vi "CRYFlatten SoundCard.vi"(11 "SoundCard":T1={"Name"="", "Analog I/O"=0, "Digital I/O"=0, "Channels"=2, "Dig Dev ID"=1, "N ports"=3, "Interface"=0, "Dig I/O Ports"=[{"port #"=1, "width"=8, "direction"=0}, {"port #"=2, "width"=8, "direction"=0}, {"port #"=3, "width"=8, "direction"=0}], "Interf settings"=[], "N interfs"=3, "udev SNs"=[], "udev enable"=FALSE, "Channel Array"=[], "Cal sequence"="", "SelectedIn"=0, "SelectedOut"=0, "SelectedTab"=0, "State"=FALSE, "Help"="", "Advanced"=FALSE, "In Audio Driver"=0, "Out Audio Driver"=0} {"Channel Array"."Coupling" items=["Default"=-1, "RSE"=10083, "NRSE"=10078, "Differential"=10106, "Pseudodifferential"=12529]; "Channel Array"."term config" items=["Default"=-1, "RSE"=10083, "NRSE"=10078, "Differential"=10106, "Pseudodifferential"=12529]; "Channel Array"."Anti-aliasing Factor (%fs)" format="%.2f"}) -> (3 "SoundCard flattened":string)   [LabVIEW 2013]
uses:
  Typedef Control/CRYHardware.ctl
  Typedef Control/CRYHardware Channel Info.ctl
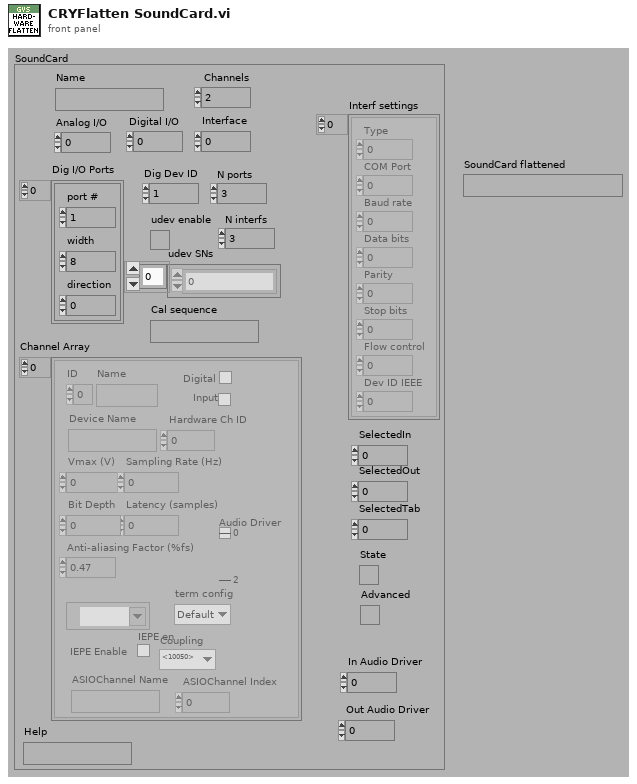
[diagram p1: front panel]
types:
  T1 = typedef "CRYHardware.ctl" = cluster{"Name":string, "Analog I/O":u16, "Digital I/O":u16, "Channels":u8, "Dig Dev ID":u8, "N ports":u8, "Interface":u32, "Dig I/O Ports":cluster{"port #":i16, "width":i16, "direction":i32}[], "Interf settings":cluster{"Type":u16, "COM Port":u8, "Baud rate":u32, "Data bits":u32, "Parity":u16, "Stop bits":u16, "Flow control":u16, "Dev ID IEEE":u8}[], "N interfs":i32, "udev SNs":i16[], "udev enable":bool, "Channel Array":T2[], "Cal sequence":string, "SelectedIn":u16, "SelectedOut":u16, "SelectedTab":u16, "State":bool, "Help":string, "Advanced":bool, "In Audio Driver":u16, "Out Audio Driver":u16}
  T2 = typedef "CRYHardware Channel Info.ctl" = cluster{"ID":i32, "Name":string, "Digital":bool, "Input":bool, "Device Name":string, "Hardware Ch ID":u8, "Vmax (V)":dbl, "Latency (samples)":dbl, "Sampling Rate (Hz)":u32, "Bit Depth":u32, "Anti-aliasing Factor (%fs)":sgl, "DAQmx Channel":tag, "term config":i32, "Coupling":i32, "IEPE en":bool, "ASIOChannel Name":string, "Audio Driver":u16, "ASIOChannel Index":u8}
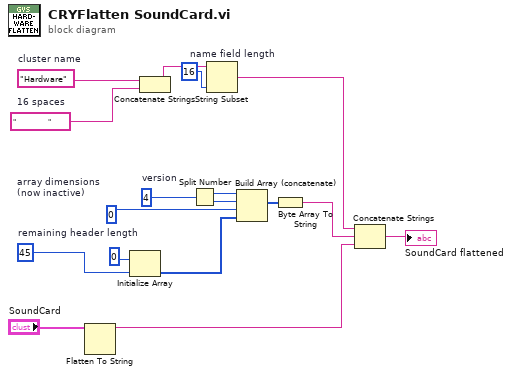
[diagram p0: block diagram]
diagram:
  w4 = u8 0  # array dimensions (now inactive)
  w7 = 16  # name field length
  w8 = "                "  # 16 spaces
  w9 = "Hardware"  # cluster name
  w13 = 45  # remaining header length
  w17 = u16 4  # version
  n1 = Flatten To String(anything="SoundCard") -> (data string=w3:string)  [unwired: 1 in, 4 out]
  n2 = Initialize Array(u8 0, w13) -> (w10:u8[])
  n3 = Concatenate Strings(w9, w8) -> (w6:string)
  n4 = Split Number(x=w17) -> (hi(x)=w16:u8, lo(x)=w15:u8)
  n5 = String Subset(string=w6, length (rest)=w7) -> (substring=w5:string)  [unwired: 1 out]
  n6 = Build Array (concatenate)(w16, w15, w4, w10) -> (w12:u8[])
  n7 = Byte Array To String(unsigned byte array=w12) -> (string=w11:string)
  n8 = Concatenate Strings(w5, w11, w3) -> (→"SoundCard flattened":string)
